vi "Write Element of Start Trigger Source.vi"(8 "error in (no error)":errorcluster, 9 "Trigger Source (None)":string(combo) caption="trigger source (None)", 10 "index":i32, 11 "CS++FgenChannelData in":refnum<class "CS++FgenChannelData.lvclass">) -> (0 "error out":errorcluster, 3 "CS++FgenChannelData out":refnum<class "CS++FgenChannelData.lvclass">)   [LabVIEW 2013, in "CS++FgenGui.lvlib" / "CS++FgenChannelData.lvclass"]
uses:
  CS++FgenChannelData.lvclass
  CS++FgenChannelData.lvclass/CS++FgenChannelData.ctl
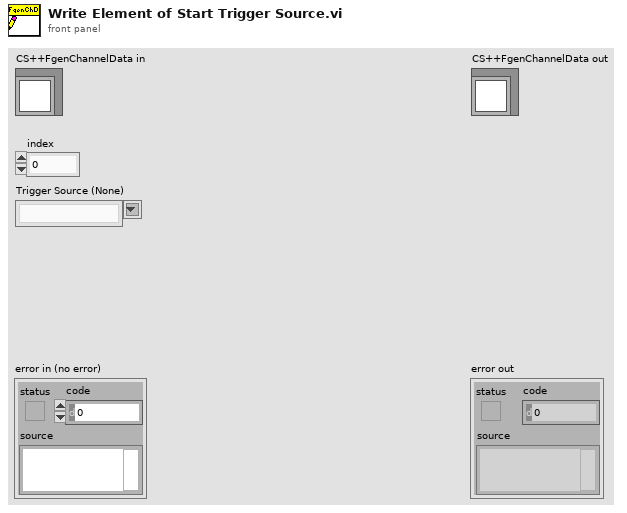
[diagram p1: front panel]
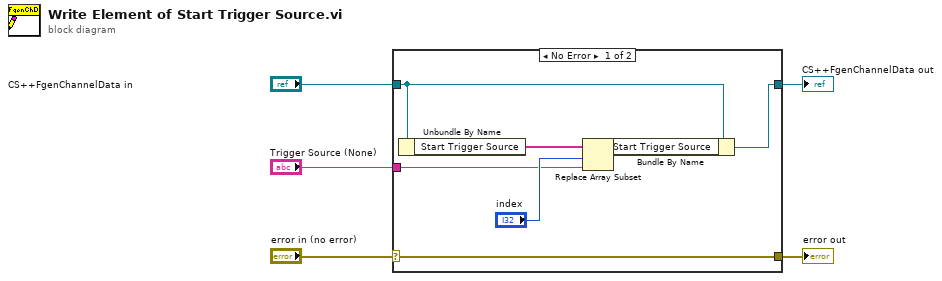
[diagram p0: block diagram]
diagram:
  n1 = case shown="No Error" "error in (no error)" {
    selector: "error in (no error)" -> [w12 w13]
    tunnel: [w12 w13] -> w4
    tunnel: [w11 w14] -> w2
    tunnel: "CS++FgenChannelData in" -> [w10 w14]
    tunnel: "Trigger Source (None)" -> [w6 _]
    frame No Error {
      n2 = Unbundle By Name(w10) -> ("Start Trigger Source"=w9:string[])
      n3 = Replace Array Subset(array=w9, new element=w6, index="index") -> (w8:string[])
      n4 = Bundle By Name(cluster=w10, "Start Trigger Source"=w8) -> (w11:refnum<class "CS++FgenChannelData.lvclass">)
    }
    frame Error {
    }
  }
  "error out" <- w4
  "CS++FgenChannelData out" <- w2
